vi "Fetch Single Record Multiple Channel(DBL).vi"(5 "FIFO Type":T1=enum."Fast FIFO", 7 "Timeout (s)":i32=5, 8 "error in":errorcluster, 11 "FPGA VI Reference In":refnum<k20>) -> (0 "error out":errorcluster, 2 "Acquired Data":dbl[][](array[numeric]) format="%.2f", 3 "FPGA VI Reference Out":refnum<k20>)   [LabVIEW 2012]
uses:
  <userlib>/FlexRIO Host Library/FlexRIO Host API/Acquire/FIFO Type.ctl
  <userlib>/FlexRIO Host Library/FlexRIO Host API/Acquire/Fetch/Fetch Acquired Data (I16).vi
  <vilib>/Utility/error.llb/Error Cluster From Error Code.vi
  <vilib>/rvi/errors/niLvFpgaAdjustHostInterfaceError.vi
  <vilib>/rvi/interface/nirviReadWriteControl/nirviReadWriteControl.xnode
  NiFpgaLv.dll
  <vilib>/rvi/interface/Simulation/niFpgaSimulationCallBeginRW.vi
  <userlib>/FlexRIO Host Library/FlexRIO Host Library (User).lvlib
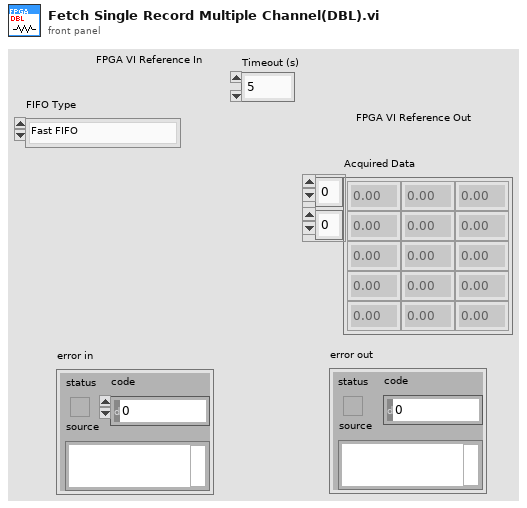
[diagram p1: front panel]
types:
  T1 = typedef "FIFO Type.ctl" = enum16{"FPGA to Host FIFO (U64)", "Generic", "FPGA to Host FIFO (U32)", "Fast FIFO"}
  T2 = cluster{"Load Record Parameters?":bool, "Pre Trigger Samples":u16, "Samples per Record":u16, "Trigger Hold Off":u16, "Record Count":u16}
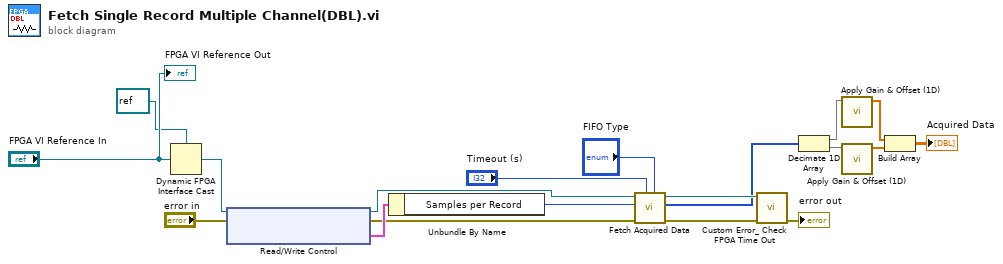
[diagram p0: block diagram]
diagram:
  n1 = Dynamic FPGA Interface Cast(Session In=refnum<k20> refnum ("Type"), Type="FPGA VI Reference In") -> (Session Out=w16:refnum<k20>)
  n2 = xnode "Read/Write Control"("FPGA VI Reference In"=w16, "error in"="error in") -> ("FPGA VI Reference Out"=w13:refnum<k20>, "error out"=w12:errorcluster, "Record Parameters"=w15:T2)
  n3 = Unbundle By Name(w15) -> ("Samples per Record"=w14:u16)
  n4 = call-poly <userlib>:"Fetch Acquired Data.vi"("FIFO Type"="FIFO Type", "Timeout (s)"="Timeout (s)", "error out"=w12, "Samples"=w14, "FPGA Reference In"=w13) -> ("error out"=w8:errorcluster, "Data"=w1:i16[], "FPGA Reference Out"=w9:refnum<k20>)  [unwired: 3 in, 1 out]
  n5 = call <userlib>:"Custom Error_ Check FPGA Time Out.vi"("error in"=w8, "FPGA VI Reference In"=w9) -> ("error out"=→"error out":errorcluster)  [unwired: 8 in, 1 out]
  n6 = Decimate 1D Array(w1) -> (w6:i16[], w3:i16[])
  n7 = call <userlib>:"Apply Gain & Offset (1D).vi"("Raw Data"=w6) -> ("Scaled Data"=w5:dbl[])  [unwired: 10 in]
  n8 = call <userlib>:"Apply Gain & Offset (1D).vi"("Raw Data"=w3) -> ("Scaled Data"=w4:dbl[])  [unwired: 10 in]
  n9 = Build Array(w5, w4) -> (→"Acquired Data":dbl[][])
  "FPGA VI Reference Out" <- "FPGA VI Reference In"
